vi "FaceDetect_SubVI.vi"(8 "error in (no error)":errorcluster, 11 "image":T1) -> (0 "error out":errorcluster, 3 "image out":T1)   [LabVIEW 2017]
uses:
  IMAQCV/Support/IMAQCV Image.ctl
  IMAQCV/IMAQCV.lvlib
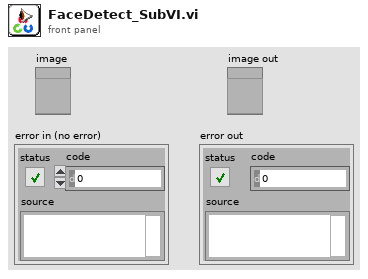
[diagram p1: front panel]
types:
  T1 = typedef "IMAQCV.lvlib/IMAQCV Image.ctl" = refnum<vi>
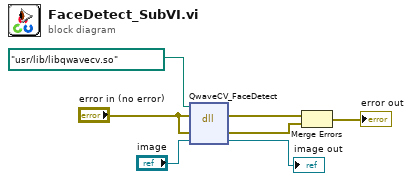
[diagram p0: block diagram]
diagram:
  n1 = dll-call lib="libqwavecv.so" fn="QwaveCV_FaceDetect"(path in=path "/usr/lib/libqwavecv.so" ("libqwaveopencv"), error in="error in (no error)", "error"="error in (no error)", "image"="image") -> (error out=w4:errorcluster, "error"=w3:errorcluster, "image"=→"image out":T1)  [unwired: 2 in, 1 out]
  n2 = Merge Errors(w4, w3) -> (→"error out":errorcluster)
